vi "FPGA Read T2H FIFO Address by Index.vi"(8 "error in (no error)":errorcluster, 9 "index":i32, 10 "Data Type":T1, 11 "FPGA Interface Base in":refnum<class "FPGA Interface Base.lvclass">) -> (0 "error out":errorcluster, 1 "Found?":bool, 2 "Address":u32, 3 "FPGA Interface Base out":refnum<class "FPGA Interface Base.lvclass">)   [LabVIEW 2010, in "FPGA Interface Base.lvclass"]
uses:
  <userlib>/_FPGA Interface Advanced Tools/FPGA Interface Base/FPGA Interface Base.lvclass
  <vilib>/rvi/DataTransferAndStorage/Container/Common/niFpgaDataTypeControl.ctl
  <userlib>/_FPGA Interface Advanced Tools/FPGA Interface Base/FPGA Interface Base.lvclass/FPGA Interface Base.ctl
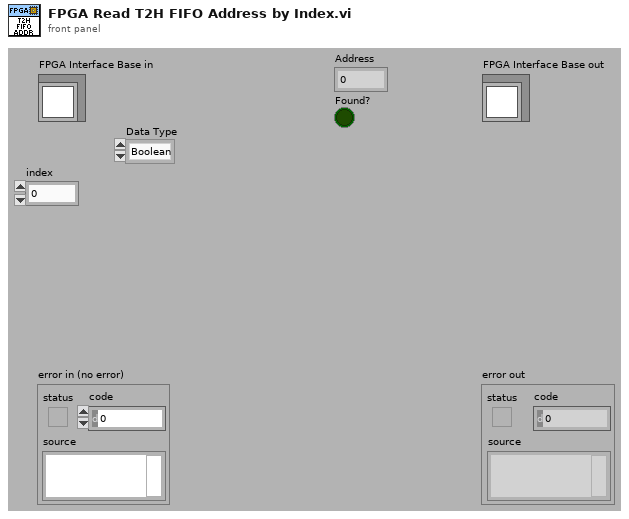
[diagram p1: front panel]
types:
  T1 = typedef "niFpgaDataTypeControl.ctl" = enum32{"Boolean", "I8", "I16", "I32", "I64", "U8", "U16", "U32", "U64", "FXP", "CustomControl"}
  T2 = typedef "FPGA Interface Base.lvclass/FPGA Session.ctl" = refnum<data-value>
  T3 = typedef "FPGA Interface Base.lvclass/FPGA Session Data.ctl" = cluster{"Session Out":u32, "Indicator Scalars":T4, "Indicator Arrays":T6, "Control Scalars":T4, "Control Arrays":T6, "TargetToHost FIFO Channels":T8, "HostToTarget FIFO Channels":T8, "All FIFOs":T9[], "IRQ Context Queue":refnum<queue>}
  T4 = typedef "FPGA Bitfile Utility.lvlib/Scalar Register Set.ctl" = cluster{"Boolean":T5[], "I8":T5[], "I16":T5[], "I32":T5[], "I64":T5[], "U8":T5[], "U16":T5[], "U32":T5[], "U64":T5[]}
  T5 = typedef "FPGA Bitfile Utility.lvlib/Scalar Register.ctl" = cluster{"Address":u32, "Name":string}
  T6 = typedef "FPGA Bitfile Utility.lvlib/Array Register Set.ctl" = cluster{"Boolean":T7[], "I8":T7[], "I16":T7[], "I32":T7[], "I64":T7[], "U8":T7[], "U16":T7[], "U32":T7[], "U64":T7[]}
  T7 = typedef "FPGA Bitfile Utility.lvlib/Array Register.ctl" = cluster{"Address":u32, "Num Elements":u32, "Name":string}
  T8 = typedef "FPGA Bitfile Utility.lvlib/FIFO Channel Set.ctl" = cluster{"Boolean":T9[], "I8":T9[], "I16":T9[], "I32":T9[], "I64":T9[], "U8":T9[], "U16":T9[], "U32":T9[], "U64":T9[]}
  T9 = typedef "FPGA Bitfile Utility.lvlib/FIFO Channel.ctl" = cluster{"Physical Channel":u32, "Name":string}
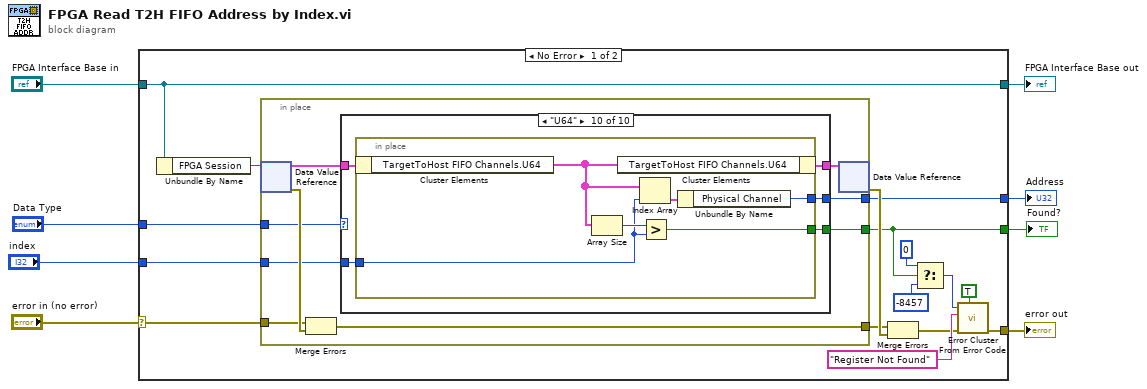
[diagram p0: block diagram]
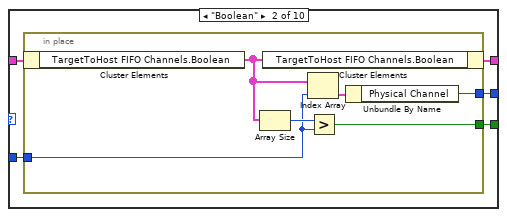
[diagram p3: hidden frame]
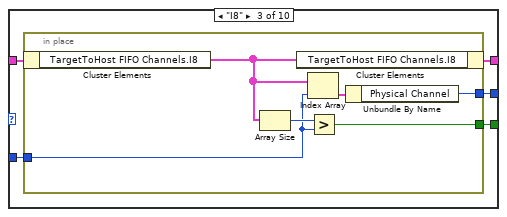
[diagram p4: hidden frame]
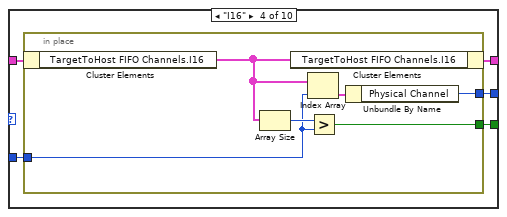
[diagram p5: hidden frame]
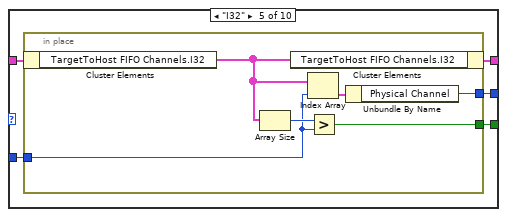
[diagram p6: hidden frame]
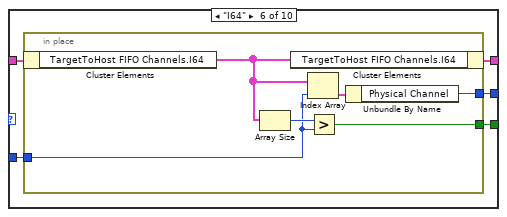
[diagram p7: hidden frame]
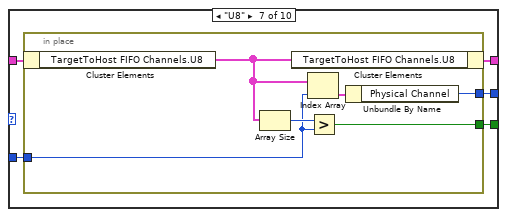
[diagram p8: hidden frame]
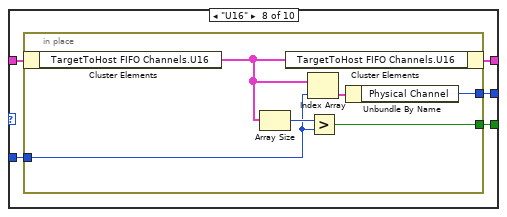
[diagram p9: hidden frame]
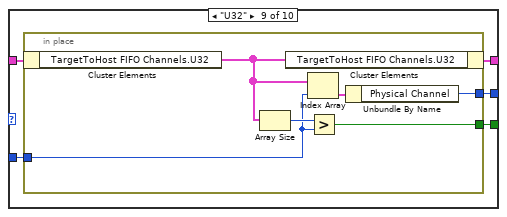
[diagram p10: hidden frame]
diagram:
  n1 = case shown="No Error" "error in (no error)" {
    selector: "error in (no error)" -> [w19 w134]
    tunnel: [w10 w134] -> w7
    tunnel: [w24 w135] -> w5
    tunnel: "FPGA Interface Base in" -> [w24 w135]
    tunnel: [w20 _] -> w4
    tunnel: [w9 _] -> w3
    tunnel: "Data Type" -> [w18 _]
    tunnel: "index" -> [w17 _]
    frame No Error {
      n2 = Unbundle By Name(w24) -> ("FPGA Session"=w21:T2)
      n3 = in-place {
        in-place-border: [w30] -> w20
        in-place-border: [w29] -> w9
        in-place-border: [w28] -> w22
        in-place-border: w19 -> [w27]
        in-place-border: w18 -> [w26]
        in-place-border: w17 -> [w25]
        n4 = in-place-dvr #1(w21) -> (w32:T3, w33:errorcluster)
        n5 = Merge Errors(w27, w33) -> (w28:errorcluster)
        n6 = case shown="\"U64\"" w26 {
          tunnel: w32 -> [w34 w39 w50 w61 w72 w83 w94 w105 w116 w127]
          tunnel: [w34 w38 w49 w60 w71 w82 w93 w104 w115 w126] -> w31
          tunnel: [_ w37 w48 w59 w70 w81 w92 w103 w114 w125] -> w30
          tunnel: [_ w36 w47 w58 w69 w80 w91 w102 w113 w124] -> w29
          tunnel: w25 -> [_ w35 w46 w57 w68 w79 w90 w101 w112 w123]
          frame Default {
          }
          frame "Boolean" {
            n7 = in-place {
              in-place-border: [w45] -> w37
              in-place-border: [w43] -> w36
              in-place-border: w35 -> [w40]
              n8 = in-place-cluster #2(w39) -> ("TargetToHost FIFO Channels.Boolean"=w42:T9[])
              n9 = Array Size(array=w42) -> (size(s)=w44:i32)
              n10 = in-place-cluster #2("TargetToHost FIFO Channels.Boolean"=w42) -> (w38:T3)
              n11 = Index Array(array=w42, index=w40) -> (element=w41:T9)
              n12 = Greater?(x=w44, y=w40) -> (0:w43:bool)
              n13 = Unbundle By Name(w41) -> ("Physical Channel"=w45:u32)
            }
          }
          frame "I8" {
            n14 = in-place {
              in-place-border: [w56] -> w48
              in-place-border: [w54] -> w47
              in-place-border: w46 -> [w51]
              n15 = in-place-cluster #3(w50) -> ("TargetToHost FIFO Channels.I8"=w53:T9[])
              n16 = Array Size(array=w53) -> (size(s)=w55:i32)
              n17 = in-place-cluster #3("TargetToHost FIFO Channels.I8"=w53) -> (w49:T3)
              n18 = Index Array(array=w53, index=w51) -> (element=w52:T9)
              n19 = Greater?(x=w55, y=w51) -> (0:w54:bool)
              n20 = Unbundle By Name(w52) -> ("Physical Channel"=w56:u32)
            }
          }
          frame "I16" {
            n21 = in-place {
              in-place-border: [w67] -> w59
              in-place-border: [w65] -> w58
              in-place-border: w57 -> [w62]
              n22 = in-place-cluster #4(w61) -> ("TargetToHost FIFO Channels.I16"=w64:T9[])
              n23 = Array Size(array=w64) -> (size(s)=w66:i32)
              n24 = in-place-cluster #4("TargetToHost FIFO Channels.I16"=w64) -> (w60:T3)
              n25 = Index Array(array=w64, index=w62) -> (element=w63:T9)
              n26 = Greater?(x=w66, y=w62) -> (0:w65:bool)
              n27 = Unbundle By Name(w63) -> ("Physical Channel"=w67:u32)
            }
          }
          frame "I32" {
            n28 = in-place {
              in-place-border: [w78] -> w70
              in-place-border: [w76] -> w69
              in-place-border: w68 -> [w73]
              n29 = in-place-cluster #5(w72) -> ("TargetToHost FIFO Channels.I32"=w75:T9[])
              n30 = Array Size(array=w75) -> (size(s)=w77:i32)
              n31 = in-place-cluster #5("TargetToHost FIFO Channels.I32"=w75) -> (w71:T3)
              n32 = Index Array(array=w75, index=w73) -> (element=w74:T9)
              n33 = Greater?(x=w77, y=w73) -> (0:w76:bool)
              n34 = Unbundle By Name(w74) -> ("Physical Channel"=w78:u32)
            }
          }
          frame "I64" {
            n35 = in-place {
              in-place-border: [w89] -> w81
              in-place-border: [w87] -> w80
              in-place-border: w79 -> [w84]
              n36 = in-place-cluster #6(w83) -> ("TargetToHost FIFO Channels.I64"=w86:T9[])
              n37 = Array Size(array=w86) -> (size(s)=w88:i32)
              n38 = in-place-cluster #6("TargetToHost FIFO Channels.I64"=w86) -> (w82:T3)
              n39 = Index Array(array=w86, index=w84) -> (element=w85:T9)
              n40 = Greater?(x=w88, y=w84) -> (0:w87:bool)
              n41 = Unbundle By Name(w85) -> ("Physical Channel"=w89:u32)
            }
          }
          frame "U8" {
            n42 = in-place {
              in-place-border: [w100] -> w92
              in-place-border: [w98] -> w91
              in-place-border: w90 -> [w95]
              n43 = in-place-cluster #7(w94) -> ("TargetToHost FIFO Channels.U8"=w97:T9[])
              n44 = Array Size(array=w97) -> (size(s)=w99:i32)
              n45 = in-place-cluster #7("TargetToHost FIFO Channels.U8"=w97) -> (w93:T3)
              n46 = Index Array(array=w97, index=w95) -> (element=w96:T9)
              n47 = Greater?(x=w99, y=w95) -> (0:w98:bool)
              n48 = Unbundle By Name(w96) -> ("Physical Channel"=w100:u32)
            }
          }
          frame "U16" {
            n49 = in-place {
              in-place-border: [w111] -> w103
              in-place-border: [w109] -> w102
              in-place-border: w101 -> [w106]
              n50 = in-place-cluster #8(w105) -> ("TargetToHost FIFO Channels.U16"=w108:T9[])
              n51 = Array Size(array=w108) -> (size(s)=w110:i32)
              n52 = in-place-cluster #8("TargetToHost FIFO Channels.U16"=w108) -> (w104:T3)
              n53 = Index Array(array=w108, index=w106) -> (element=w107:T9)
              n54 = Greater?(x=w110, y=w106) -> (0:w109:bool)
              n55 = Unbundle By Name(w107) -> ("Physical Channel"=w111:u32)
            }
          }
          frame "U32" {
            n56 = in-place {
              in-place-border: [w122] -> w114
              in-place-border: [w120] -> w113
              in-place-border: w112 -> [w117]
              n57 = in-place-cluster #9(w116) -> ("TargetToHost FIFO Channels.U32"=w119:T9[])
              n58 = Array Size(array=w119) -> (size(s)=w121:i32)
              n59 = in-place-cluster #9("TargetToHost FIFO Channels.U32"=w119) -> (w115:T3)
              n60 = Index Array(array=w119, index=w117) -> (element=w118:T9)
              n61 = Greater?(x=w121, y=w117) -> (0:w120:bool)
              n62 = Unbundle By Name(w118) -> ("Physical Channel"=w122:u32)
            }
          }
          frame "U64" {
            n63 = in-place {
              in-place-border: [w133] -> w125
              in-place-border: [w131] -> w124
              in-place-border: w123 -> [w128]
              n64 = in-place-cluster #10(w127) -> ("TargetToHost FIFO Channels.U64"=w130:T9[])
              n65 = Array Size(array=w130) -> (size(s)=w132:i32)
              n66 = in-place-cluster #10("TargetToHost FIFO Channels.U64"=w130) -> (w126:T3)
              n67 = Index Array(array=w130, index=w128) -> (element=w129:T9)
              n68 = Greater?(x=w132, y=w128) -> (0:w131:bool)
              n69 = Unbundle By Name(w129) -> ("Physical Channel"=w133:u32)
            }
          }
        }
        n70 = in-place-dvr #1(w31) -> (w23:errorcluster)  [unwired: 1 out]
      }
      n71 = Merge Errors(w22, w23) -> (w11:errorcluster)
      n72 = Select(t=0, s=w9, f=-8457 ("error code (0)")) -> (s? t:f=w15:i32)
      n73 = call <vilib>:"Error Cluster From Error Code.vi"("show call chain? (False)"=TRUE, "error in (no error)"=w11, "error message (\"\")"="Register Not Found" ("string"), "error code (0)"=w15) -> ("error out"=w10:errorcluster)  [unwired: 5 in]
    }
    frame Error {
    }
  }
  "error out" <- w7
  "FPGA Interface Base out" <- w5
  "Address" <- w4
  "Found?" <- w3
